vi "My JKI State Machine Module.vi"(7 "Module Name":string="M1") -> ()   [LabVIEW 2017, in "CSM Example echo DQMH.lvlib"]
doc: "------------- lvcsm -------------\n[CSMStates]\nItem 0 = \"Event Structure\"\nItem 1 = \"Idle\"\nItem 2 = \"Target Timeout Error\"\nItem 3 = \"Target Error\"\nItem 4 = \"Initialize Core Data\"\nItem 5 = \"VI Reference\"\nItem 6 = \"Error Handler\"\nItem 7 = \"Exit\"\nItem 8 = \"Data: Initialize\"\nItem 9 = \"Data: Cleanup\"\nItem 10 = \"UI: Initialize\"\nItem 11 = \"UI: Cursor Set\"\nItem 12 = \"UI: Front Panel State\"\nItem 13 = \"Macro: Initialize\"\nItem 14 = \"Macro: Exit\"\nItem 15 = \"New Category: 1\"\nItem 16 = \"New Category: 2\"\nItem 17 = \"Test: Do Something\"\nItem 18 = \"Test: Do Something Else\"\nItem 19 = \"Test: Do Something Else and Wait for Reply\"\n\n[CSMStatus]\nItem 0 = \"Test: Do Something Else@Event Structure\"\nItem 1 = \"Test: Do Something Else@Idle\""
uses:
  CSM Example echo DQMH.lvlib
  <vilib>/ErrorRing/Error Ring.xnode
  user.lib/_NEVSTOP/Communicable State Machine(CSM)/Communicable State Machine.lvlib
panel:
  out "Status":string
  out "error out":errorcluster
  in  "Simulate  Error":bool
  out "X":dbl
  in  "Do Something Else <Replace Me>":bool
  in  "Do Something <Replace Me>":bool
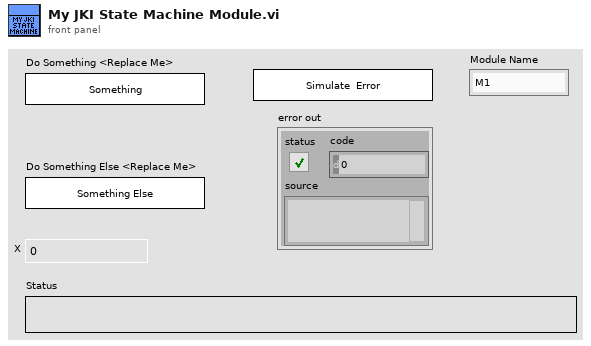
[diagram p1: front panel]
types:
  T1 = enum32{"Invalid", "Standard", "Closed", "Hidden", "Minimized", "Maximized"}
  T2 = enum32{"invalid app kind", "Development System", "Run Time System", "Student Edition", "Embedded LabVIEW", "Evaluation", "Custom"}
  T3 = cluster{"Core":cluster{"Current VI Reference":refnum<vi>, "Close Panel on Exit?":bool}, "Your Boolean data":bool, "Your string data":string}
  T4 = cluster{"Current VI Reference":refnum<vi>, "Close Panel on Exit?":bool}
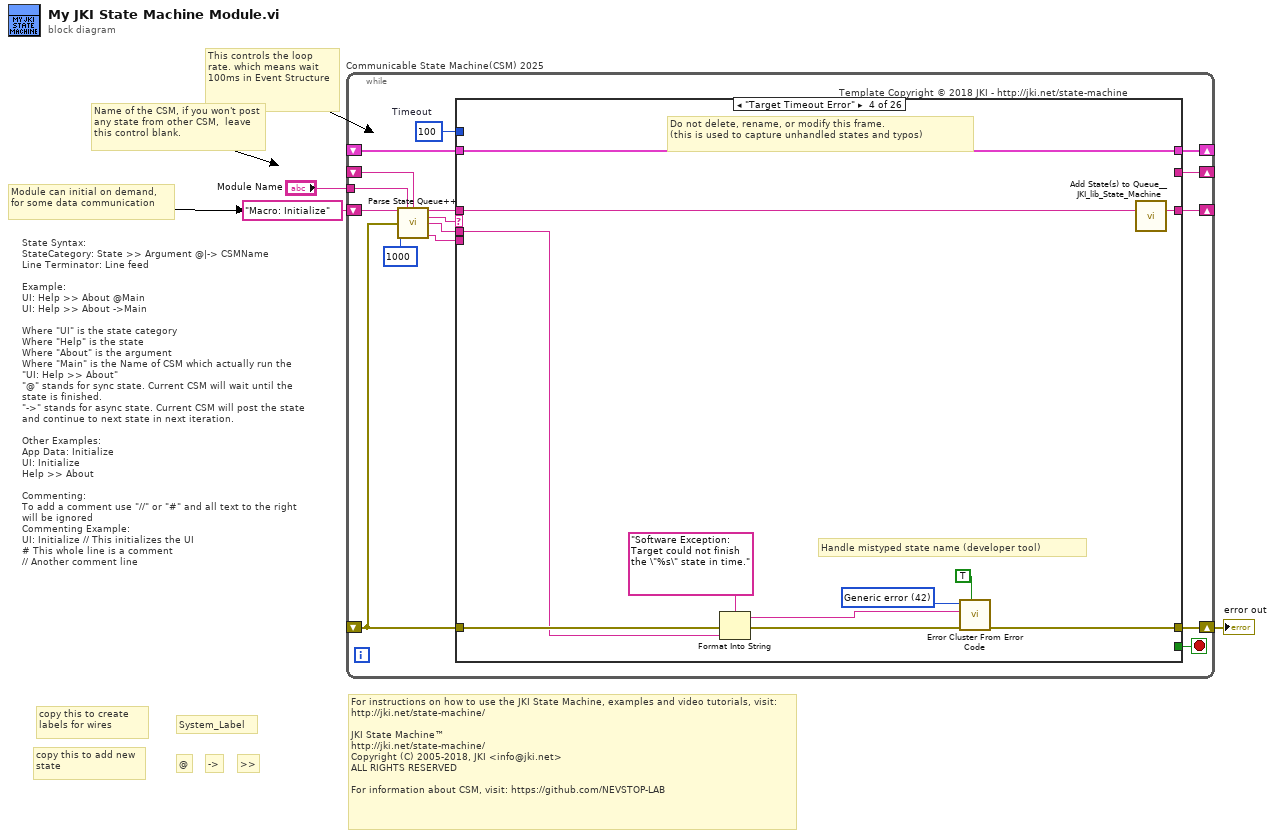
[diagram p0: block diagram]
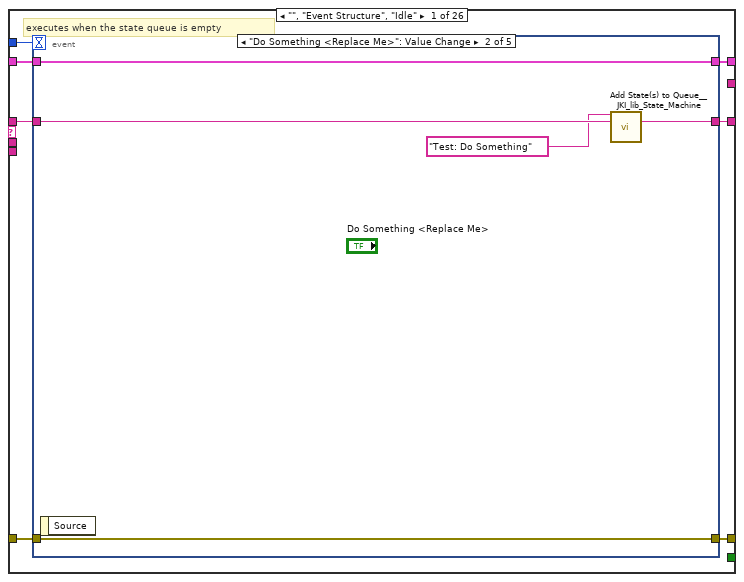
[diagram p2: hidden frame]
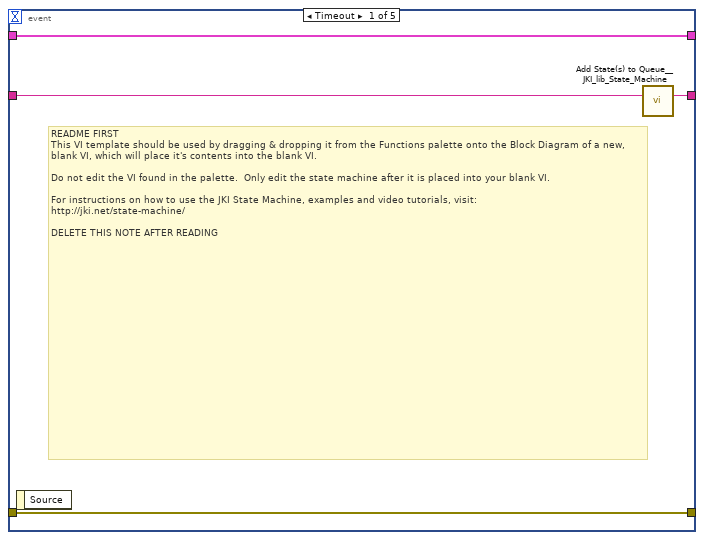
[diagram p3: hidden frame]
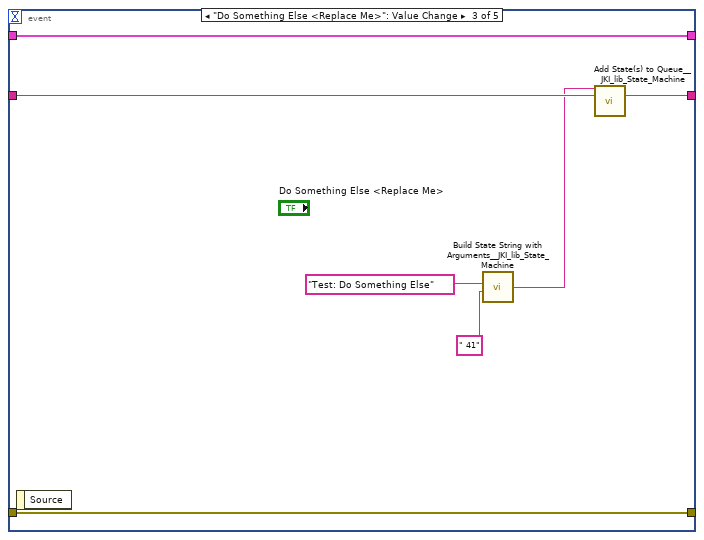
[diagram p4: hidden frame]
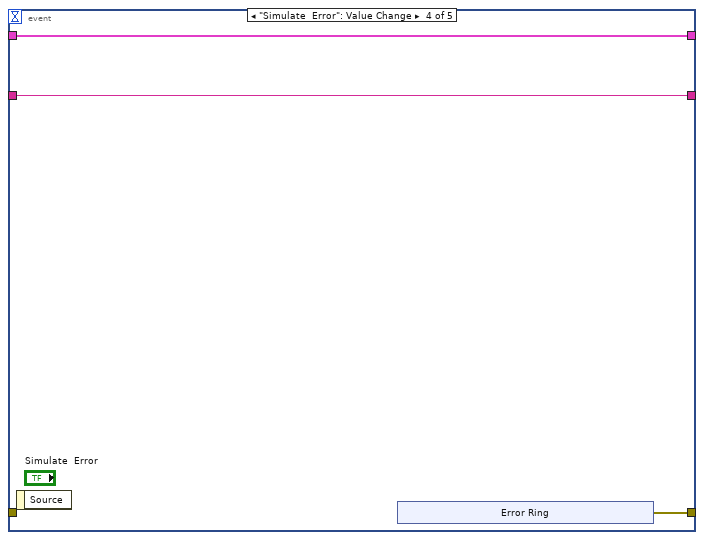
[diagram p5: hidden frame]
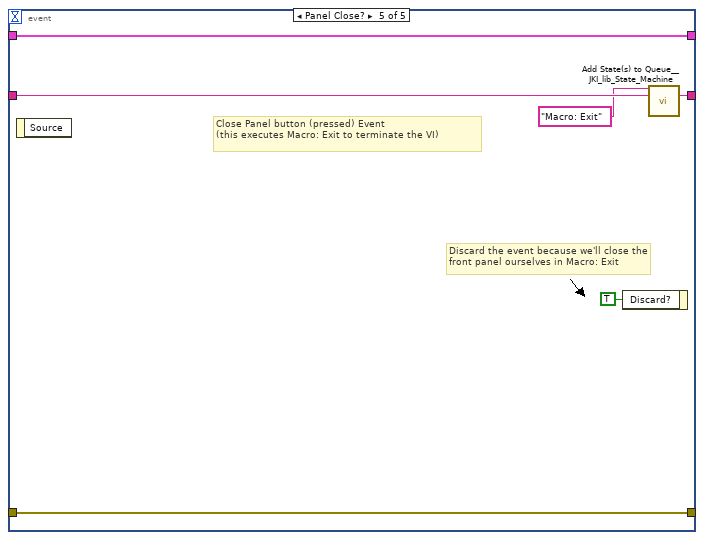
[diagram p6: hidden frame]
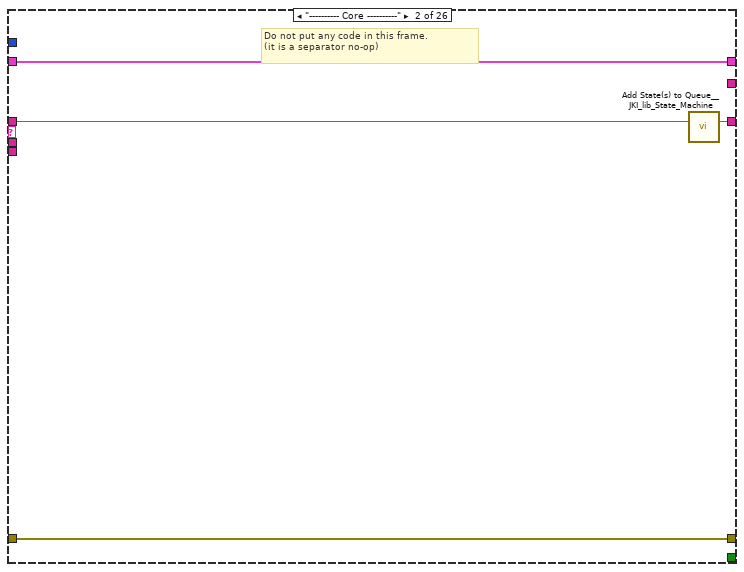
[diagram p7: hidden frame]
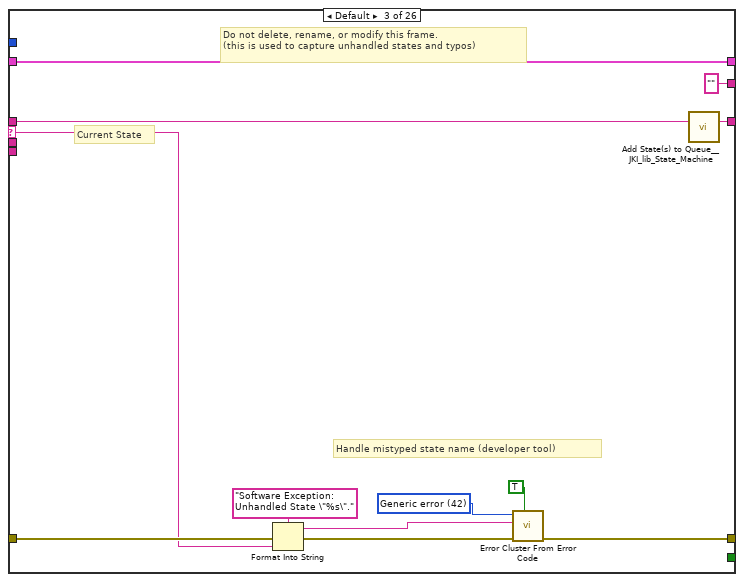
[diagram p8: hidden frame]
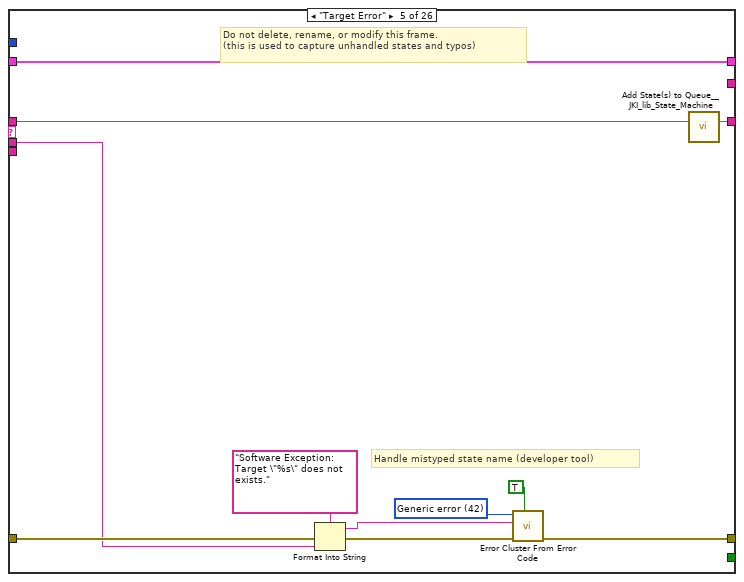
[diagram p9: hidden frame]
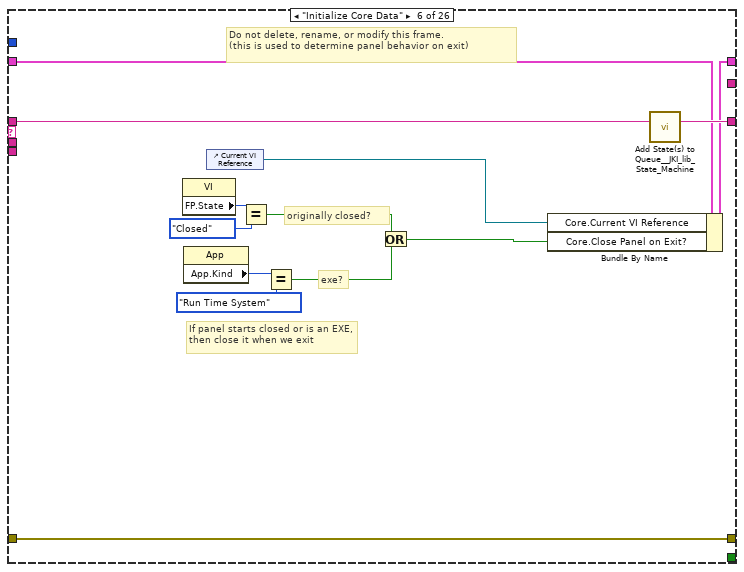
[diagram p10: hidden frame]
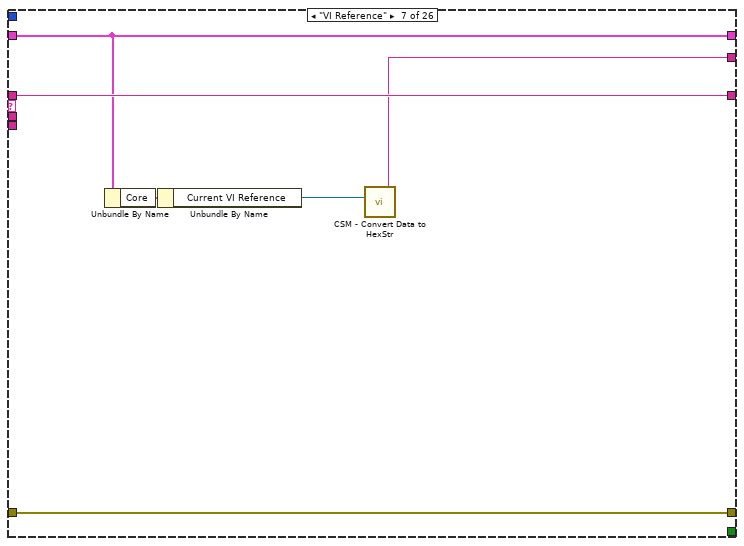
[diagram p11: hidden frame]
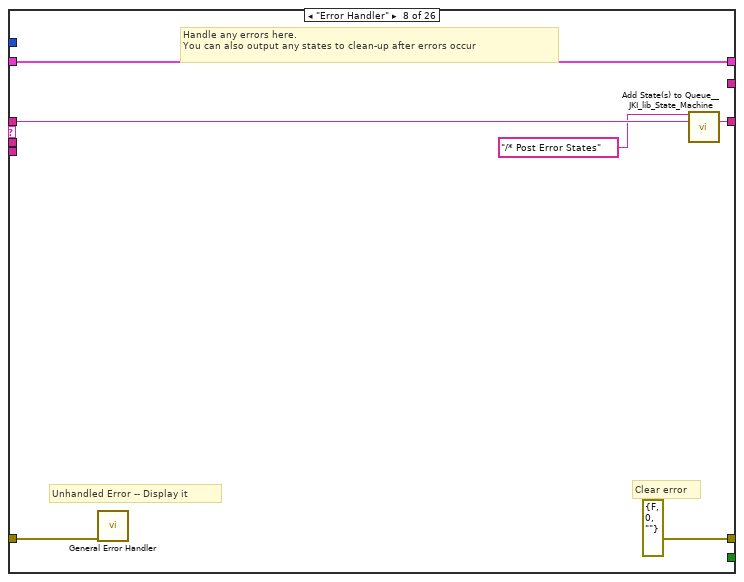
[diagram p12: hidden frame]
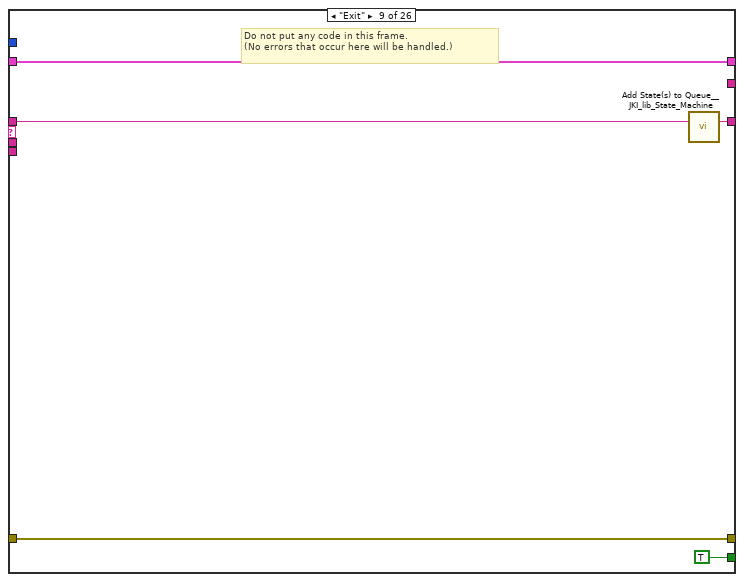
[diagram p13: hidden frame]
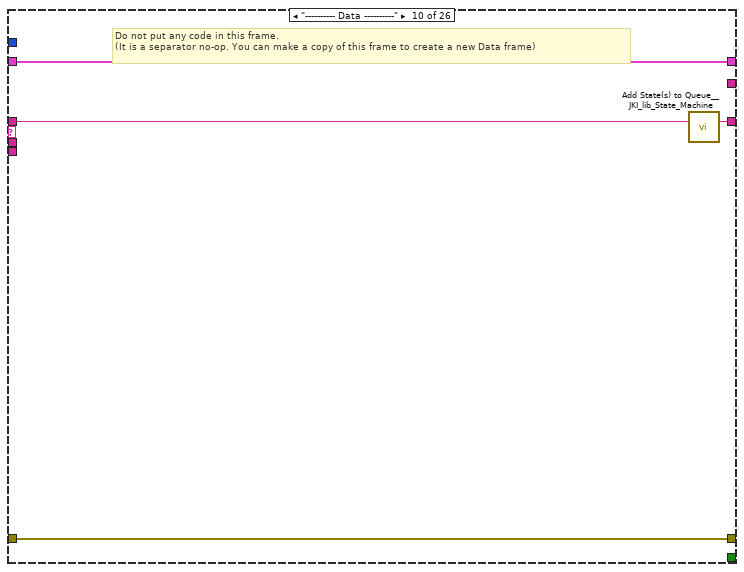
[diagram p14: hidden frame]
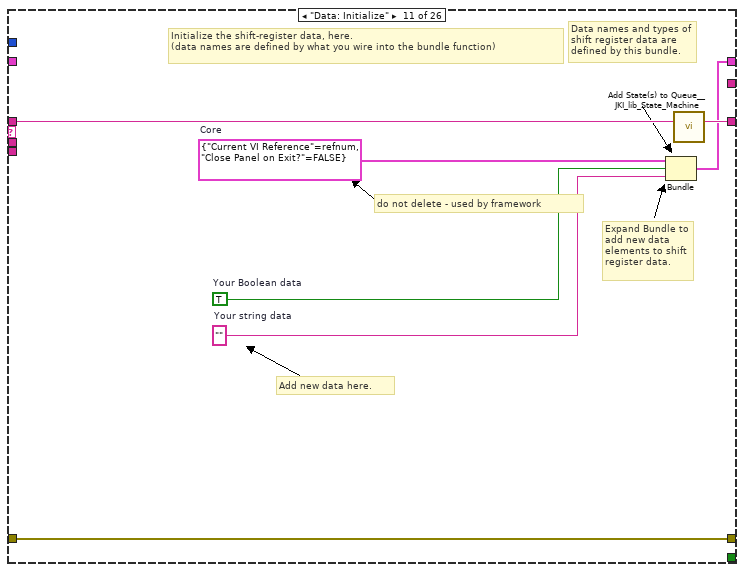
[diagram p15: hidden frame]
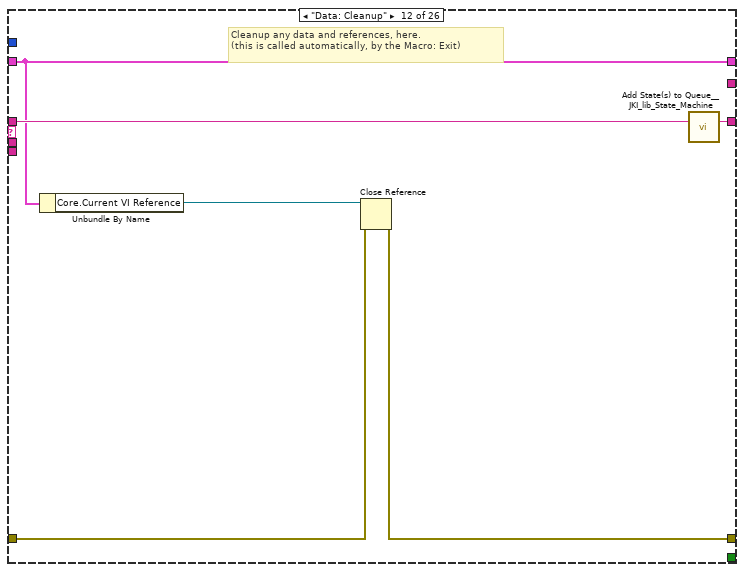
[diagram p16: hidden frame]
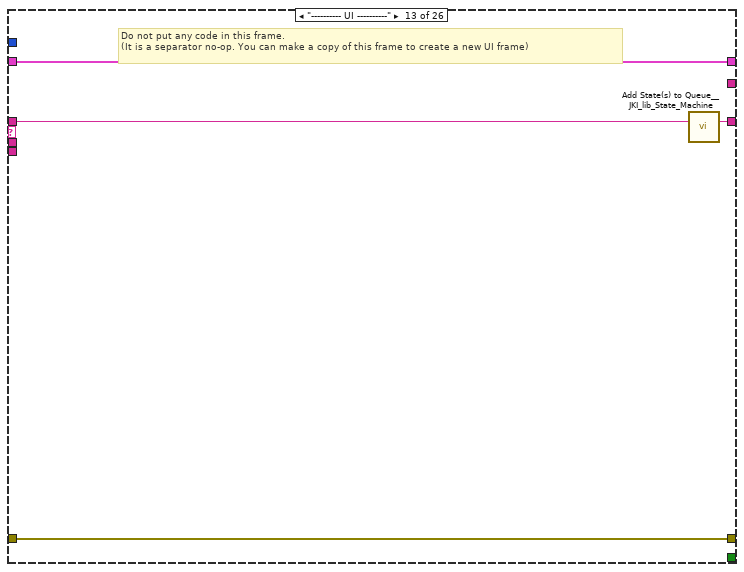
[diagram p17: hidden frame]
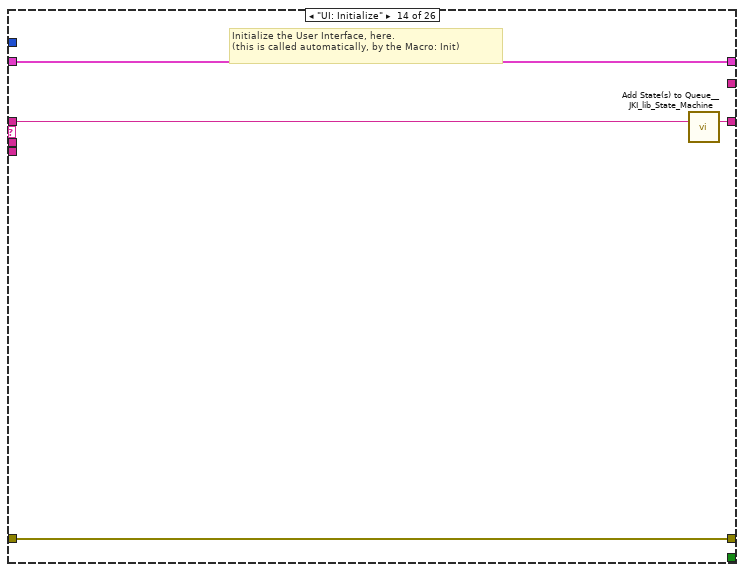
[diagram p18: hidden frame]
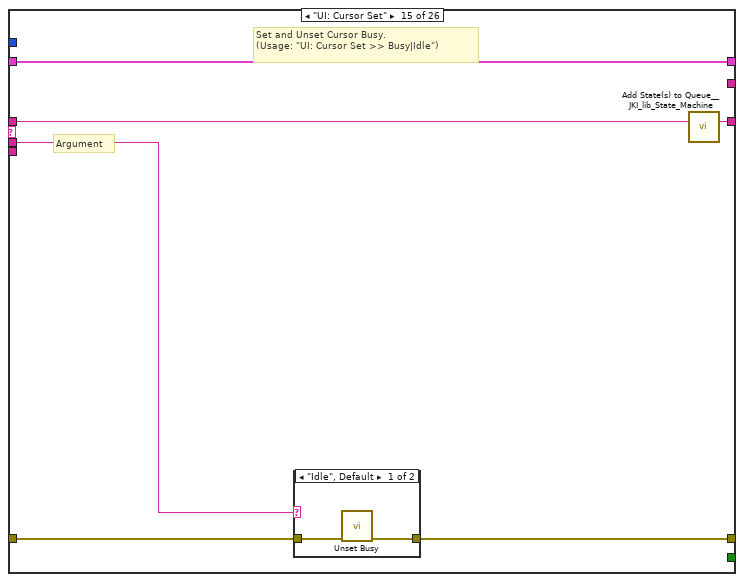
[diagram p19: hidden frame]
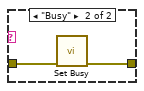
[diagram p20: hidden frame]
diagram:
  # "For instructions on how to use the JKI State Machine, examples and video tutorials, visit: http://jki.net/state-machine/\n\nJKI State Machine™\nhttp://jki.net/state-machine/\nCopyright (C) 2005-2018, JKI <info@jki.net>\nALL RIGHTS RESERVED\n\nFor information about CSM, visit: https://github.com/NEVSTOP-LAB"
  # "copy this to add new state"
  # ">>"
  # "->"
  # "@"
  # "State Syntax:\nStateCategory: State >> Argument @|-> CSMName\nLine Terminator: Line feed\n\nExample:\nUI: Help >> About @Main\nUI: Help >> About ->Main\n\nWhere \"UI\" is the state category\nWhere \"Help\" is the state\nWhere \"About\" is the argument\nWhere \"Main\" is the Name of CSM which actually run the \"UI: Help >> About\"\n\"@\" stands for sync state. Current CSM will wait until the state is finished.\n\"->\" stands for async state. Current CSM will post the state and continue to next state in next iteration.\n\nOther Examples:\nApp Data: Initialize\nUI: Initialize\nHelp >> About\n\nCommenting:\nTo add a comment use \"//\" or \"#\" and all text to the right will be ignored\nCommenting Example:\nUI: Initialize // This initializes the UI\n# This whole line is a comment\n// Another comment line"
  # "copy this to create labels for wires"
  # "System_Label"
  # "Module can initial on demand,\nfor some data communication"
  # "Name of the CSM, if you won't post any state from other CSM,  leave this control blank."
  # "This controls the loop rate. which means wait 100ms in Event Structure"
  n1 = while "Communicable State Machine(CSM) 2025" {
    shift-right: [w14] -> _
    shift-left: _ -> [w13]
    shift-right: [w17] -> w1
    shift-left: _ -> [w11]
    shift-right: [w16] -> _
    shift-left: "Macro: Initialize" ("States Out") -> [w18]
    tunnel: "Module Name" -> [w7]
    shift-right: [w4] -> _
    shift-left: _ -> [w5]
    stop <- w15 stop-if-true
    w12 = 100  # Timeout
    # "Template Copyright © 2018 JKI - http://jki.net/state-machine"
    n2 = call "Parse State Queue++.vi"("State Queue"=w18, "Name (\"\" to Use UUID)"=w7, "Response Arguments"=w5, "Previous Error"=w11, "Response Timeout (-2 Use Global Settings)"=1000 ("Response Timeout(1000ms)")) -> ("Remaining States"=w19:string, "Current State"=w10:string, "Arguments"=w9:string, ">> Source CSM >>"=w8:string)  [unwired: 5 in, 2 out]
    n3 = case shown="\"Target Timeout Error\"" w10 {
      selector: w10 -> [_ _ w62 _ _ _ _ _ _ _ _ _ _ _ _ _ _ _ _ _ _ _ _ _ _ _]
      tunnel: w19 -> [w26 w60 w66 w77 w88 w107 w112 w119 w124 w128 w135 w141 w145 w149 w155 w166 w235 w240 w250 w254 w258 w262 w266 w277 w291 w307]
      tunnel: w9 -> [_ _ _ w73 w84 _ _ _ _ _ _ _ _ _ w150 w160 _ _ _ _ _ _ _ _ w281 w296]
      tunnel: w13 -> [w24 w57 w64 w75 w86 w100 w111 w116 w122 w125 _ w136 w142 w147 w153 w162 w232 w237 w247 w251 w255 w259 w263 w276 w290 w306]
      tunnel: [w23 w58 w68 w79 w90 w104 w113 errorcluster {"status"=FALSE, "code"=0, "source"=""} ("error out") w121 w126 w132 w137 w143 w146 w151 w163 w233 w238 w248 w252 w256 w260 w264 w278 w292 w308] -> w17
      tunnel: w11 -> [w22 w58 w67 w78 w89 w104 w113 w115 w121 w126 w132 w138 w143 w146 w152 w164 w233 w238 w248 w252 w256 w260 w264 w278 w292 w308]
      tunnel: [w25 w59 w65 w76 w87 w106 w112 w118 w123 w127 w134 w140 w144 w148 w154 w165 w234 w239 w249 w253 w257 w261 w265 w277 w291 w307] -> w16
      tunnel: [_ _ _ _ _ _ _ _ TRUE _ _ _ _ _ _ _ _ _ _ _ _ _ _ _ _ _] -> w15
      tunnel: [w21 w57 w64 w75 w86 w105 w111 w116 w122 w125 w133 w136 w142 w147 w153 w162 w232 w237 w247 w251 w255 w259 w263 w276 w290 w306] -> w14
      tunnel: w12 -> [w20 _ _ _ _ _ _ _ _ _ _ _ _ _ _ _ _ _ _ _ _ _ _ _ _ _]
      tunnel: w8 -> [_ _ _ _ _ _ _ _ _ _ _ _ _ _ _ _ _ _ _ _ _ _ _ w268 w283 w299]
      tunnel: [_ _ "" _ _ _ w108 _ _ _ _ _ _ _ _ _ _ _ _ _ _ _ _ w267 w279 w293] -> w4
      frame "", "Event Structure", "Idle" {
        # "executes when the state queue is empty"
        n4 = event shown="[1] \"Do Something <Replace Me>\": Value Change" {
          selector: _ -> [_ _ _ _ _]
          dyn-events: _ -> [_ _ _ _ _]
          timeout: w20 -> [_ _ _ _ _]
          tunnel: w26 -> [w30 w35 w42 w44 w56]
          tunnel: [w29 w34 w41 w44 w55] -> w25
          tunnel: w24 -> [w27 w33 w40 w45 w53]
          tunnel: [w28 w31 w39 w43 w54] -> w23
          tunnel: w22 -> [w28 w31 w39 _ w54]
          tunnel: [w27 w33 w40 w45 w53] -> w21
          event Timeout {
            # "README FIRST\nThis VI template should be used by dragging & dropping it from the Functions palette onto the Block Diagram of a new, blank VI, which will place it's contents into the blank VI.\n\nDo not edit the VI found in the palette.  Only edit the state machine after it is placed into your blank VI.\n\nFor instructions on how to use the JKI State Machine, examples and video tutorials, visit:\nhttp://jki.net/state-machine/\n\nDELETE THIS NOTE AFTER READING"
            n5 = event-data() -> ()  [unwired: 1 in, 1 out]
            n6 = call <vilib>:"Add State(s) to Queue__JKI_lib_State_Machine.vi"("State(s) in (\"\")"=w30) -> ("States Out"=w29:string)  [unwired: 14 in]
          }
          event "Do Something <Replace Me>": Value Change {
            n7 = event-data() -> ()  [unwired: 1 in, 1 out]
            n8 = call <vilib>:"Add State(s) to Queue__JKI_lib_State_Machine.vi"("State(s) in Front (\"\")"="Test: Do Something" ("State(s) in Front (\"\")"), "State(s) in (\"\")"=w35) -> ("States Out"=w34:string)  [unwired: 13 in]
          }
          event "Do Something Else <Replace Me>": Value Change {
            n9 = event-data() -> ()  [unwired: 1 in, 1 out]
            n10 = call <vilib>:"Build State String with Arguments__JKI_lib_State_Machine.vi"("Arguments (\"\")"=" 41" ("Arguments (\"\")"), "State"="Test: Do Something Else" ("State(s) in Front (\"\")")) -> ("State with Arguments"=w37:string)  [unwired: 4 in]
            n11 = call <vilib>:"Add State(s) to Queue__JKI_lib_State_Machine.vi"("State(s) in Front (\"\")"=w37, "State(s) in (\"\")"=w42) -> ("States Out"=w41:string)  [unwired: 13 in]
          }
          event "Simulate  Error": Value Change {
            n12 = event-data() -> ()  [unwired: 1 in, 1 out]
            n13 = xnode "Error Ring"() -> ("error out"=w43:errorcluster)
          }
          event Panel Close? {
            # "Discard the event because we'll close the front panel ourselves in Macro: Exit"
            # "Close Panel button (pressed) Event\n(this executes Macro: Exit to terminate the VI)"
            n14 = event-data() -> ()  [unwired: 1 in, 1 out]
            n15 = event-data("Discard?"=TRUE) -> ()  [unwired: 1 in, 1 out]
            n16 = call <vilib>:"Add State(s) to Queue__JKI_lib_State_Machine.vi"("State(s) in Front (\"\")"="Macro: Exit", "State(s) in (\"\")"=w56) -> ("States Out"=w55:string)  [unwired: 13 in]
          }
        }
      }
      frame "---------- Core ----------" {
        # "Do not put any code in this frame.\n(it is a separator no-op)"
        n17 = call <vilib>:"Add State(s) to Queue__JKI_lib_State_Machine.vi"("State(s) in (\"\")"=w60) -> ("States Out"=w59:string)  [unwired: 14 in]
      }
      frame Default {
        w71 = 42 items=["No error", "Argument error", "Memory is full", "Out of zone", "End of file", "File already open", "Generic file I/O error", "File not found", "File permission error", "Disk is full", "Duplicate path", "Too many files open", "System feature not enabled", "Resource file not found", "Cannot add resource", "Resource not found", "Image not found", "Image memory error", "Pen does not exist", "Config type invalid", "Config token not found", "Config parse error", "Config memory error", "Bad external code format", "Bad external code offset", "External code not present", "Null window", "Destroy window error", "Null menu", "Print aborted", "Bad print record", "Print driver error", "Windows error during printing", "Memory error during printing", "Print dialog error", "Generic print error", "Invalid device refnum", "Device not found", "Device parameter error", "Device unit error", "Cannot open device", "Device call aborted", "Generic error", "Cancelled by user", "Object ID too low", "Object ID too high", "Object not in heap", "Unknown heap", "Unknown object (invalid DefProc)", "Unknown object (DefProc not in table)", "Message out of range", "Invalid (null) method", "Unknown message", "Manager call not supported", "Bad address", "Network operation in progress", "Network operation timed out", "Connection is busy", "Network attribute not supported", "Network error", "Address in use", "System out of memory", "Connection aborted", "Connection refused", "Not connected", "Already connected", "Connection closed", "Initialization error (interapplication manager)", "Bad occurrence", "Wait on unbound occurrence handler", "Occurrence queue overflow", "Datalog type conflict", "Unused", "Unrecognized type (interapplication manager)", "Memory corrupt", "Failed to make temporary DLL", "Old CIN version", "Drag socket not found", "Failed to load drop-object", "Failed to register OLE object", "Failed to release OLE object", "Format specifier type mismatch", "Unknown format specifier", "Too few format specifiers", "Too many format specifiers", "Scan failed", "Newer CIN version", "Error converting to variant", "Runtime menu error", "Password tampered", "Variant attribute not found", "Incompatible variant data type", "Event data is not available", "Event Store is not present", "Occurrence is not found", "Event Queue is not created", "Event info is not available", "Refnum passed is NULL", "Error retrieving Class GUID", "Error retrieving CoClass GUID", "Error retrieving TypeLib GUID.", "Bad built application magic bytes.", "Specific driver is different from the specific driver associated with the Logical Name.", "There is no session opened to the class driver.", "Max Error", "MAX - Error with config objects", "MAX - Error loading configuration", "MAX - Group not supported"]
        # "Current State"
        # "Do not delete, rename, or modify this frame.\n(this is used to capture unhandled states and typos)"
        # "Handle mistyped state name (developer tool)"
        n18 = Format Into String(format string="Software Exception: Unhandled State \"%s\"." ("message"), error in=w67, w62) -> (resulting string=w70:string, error out=w69:errorcluster)  [unwired: 1 in]
        n19 = call <vilib>:"Error Cluster From Error Code.vi"("show call chain? (False)"=TRUE, "error in (no error)"=w69, "error message (\"\")"=w70, "error code (0)"=w71) -> ("error out"=w68:errorcluster)  [unwired: 5 in]
        n20 = call <vilib>:"Add State(s) to Queue__JKI_lib_State_Machine.vi"("State(s) in (\"\")"=w66) -> ("States Out"=w65:string)  [unwired: 14 in]
      }
      frame "Target Timeout Error" {
        w82 = 42 items=["No error", "Argument error", "Memory is full", "Out of zone", "End of file", "File already open", "Generic file I/O error", "File not found", "File permission error", "Disk is full", "Duplicate path", "Too many files open", "System feature not enabled", "Resource file not found", "Cannot add resource", "Resource not found", "Image not found", "Image memory error", "Pen does not exist", "Config type invalid", "Config token not found", "Config parse error", "Config memory error", "Bad external code format", "Bad external code offset", "External code not present", "Null window", "Destroy window error", "Null menu", "Print aborted", "Bad print record", "Print driver error", "Windows error during printing", "Memory error during printing", "Print dialog error", "Generic print error", "Invalid device refnum", "Device not found", "Device parameter error", "Device unit error", "Cannot open device", "Device call aborted", "Generic error", "Cancelled by user", "Object ID too low", "Object ID too high", "Object not in heap", "Unknown heap", "Unknown object (invalid DefProc)", "Unknown object (DefProc not in table)", "Message out of range", "Invalid (null) method", "Unknown message", "Manager call not supported", "Bad address", "Network operation in progress", "Network operation timed out", "Connection is busy", "Network attribute not supported", "Network error", "Address in use", "System out of memory", "Connection aborted", "Connection refused", "Not connected", "Already connected", "Connection closed", "Initialization error (interapplication manager)", "Bad occurrence", "Wait on unbound occurrence handler", "Occurrence queue overflow", "Datalog type conflict", "Unused", "Unrecognized type (interapplication manager)", "Memory corrupt", "Failed to make temporary DLL", "Old CIN version", "Drag socket not found", "Failed to load drop-object", "Failed to register OLE object", "Failed to release OLE object", "Format specifier type mismatch", "Unknown format specifier", "Too few format specifiers", "Too many format specifiers", "Scan failed", "Newer CIN version", "Error converting to variant", "Runtime menu error", "Password tampered", "Variant attribute not found", "Incompatible variant data type", "Event data is not available", "Event Store is not present", "Occurrence is not found", "Event Queue is not created", "Event info is not available", "Refnum passed is NULL", "Error retrieving Class GUID", "Error retrieving CoClass GUID", "Error retrieving TypeLib GUID.", "Bad built application magic bytes.", "Specific driver is different from the specific driver associated with the Logical Name.", "There is no session opened to the class driver.", "Max Error", "MAX - Error with config objects", "MAX - Error loading configuration", "MAX - Group not supported"]
        # "Do not delete, rename, or modify this frame.\n(this is used to capture unhandled states and typos)"
        # "Handle mistyped state name (developer tool)"
        n21 = Format Into String(format string="Software Exception: Target could not finish the \"%s\" state in time." ("message"), error in=w78, w73) -> (resulting string=w81:string, error out=w80:errorcluster)  [unwired: 1 in]
        n22 = call <vilib>:"Error Cluster From Error Code.vi"("show call chain? (False)"=TRUE, "error in (no error)"=w80, "error message (\"\")"=w81, "error code (0)"=w82) -> ("error out"=w79:errorcluster)  [unwired: 5 in]
        n23 = call <vilib>:"Add State(s) to Queue__JKI_lib_State_Machine.vi"("State(s) in (\"\")"=w77) -> ("States Out"=w76:string)  [unwired: 14 in]
      }
      frame "Target Error" {
        w93 = 42 items=["No error", "Argument error", "Memory is full", "Out of zone", "End of file", "File already open", "Generic file I/O error", "File not found", "File permission error", "Disk is full", "Duplicate path", "Too many files open", "System feature not enabled", "Resource file not found", "Cannot add resource", "Resource not found", "Image not found", "Image memory error", "Pen does not exist", "Config type invalid", "Config token not found", "Config parse error", "Config memory error", "Bad external code format", "Bad external code offset", "External code not present", "Null window", "Destroy window error", "Null menu", "Print aborted", "Bad print record", "Print driver error", "Windows error during printing", "Memory error during printing", "Print dialog error", "Generic print error", "Invalid device refnum", "Device not found", "Device parameter error", "Device unit error", "Cannot open device", "Device call aborted", "Generic error", "Cancelled by user", "Object ID too low", "Object ID too high", "Object not in heap", "Unknown heap", "Unknown object (invalid DefProc)", "Unknown object (DefProc not in table)", "Message out of range", "Invalid (null) method", "Unknown message", "Manager call not supported", "Bad address", "Network operation in progress", "Network operation timed out", "Connection is busy", "Network attribute not supported", "Network error", "Address in use", "System out of memory", "Connection aborted", "Connection refused", "Not connected", "Already connected", "Connection closed", "Initialization error (interapplication manager)", "Bad occurrence", "Wait on unbound occurrence handler", "Occurrence queue overflow", "Datalog type conflict", "Unused", "Unrecognized type (interapplication manager)", "Memory corrupt", "Failed to make temporary DLL", "Old CIN version", "Drag socket not found", "Failed to load drop-object", "Failed to register OLE object", "Failed to release OLE object", "Format specifier type mismatch", "Unknown format specifier", "Too few format specifiers", "Too many format specifiers", "Scan failed", "Newer CIN version", "Error converting to variant", "Runtime menu error", "Password tampered", "Variant attribute not found", "Incompatible variant data type", "Event data is not available", "Event Store is not present", "Occurrence is not found", "Event Queue is not created", "Event info is not available", "Refnum passed is NULL", "Error retrieving Class GUID", "Error retrieving CoClass GUID", "Error retrieving TypeLib GUID.", "Bad built application magic bytes.", "Specific driver is different from the specific driver associated with the Logical Name.", "There is no session opened to the class driver.", "Max Error", "MAX - Error with config objects", "MAX - Error loading configuration", "MAX - Group not supported"]
        # "Do not delete, rename, or modify this frame.\n(this is used to capture unhandled states and typos)"
        # "Handle mistyped state name (developer tool)"
        n24 = Format Into String(format string="Software Exception: Target \"%s\" does not exists." ("message"), error in=w89, w84) -> (resulting string=w92:string, error out=w91:errorcluster)  [unwired: 1 in]
        n25 = call <vilib>:"Error Cluster From Error Code.vi"("show call chain? (False)"=TRUE, "error in (no error)"=w91, "error message (\"\")"=w92, "error code (0)"=w93) -> ("error out"=w90:errorcluster)  [unwired: 5 in]
        n26 = call <vilib>:"Add State(s) to Queue__JKI_lib_State_Machine.vi"("State(s) in (\"\")"=w88) -> ("States Out"=w87:string)  [unwired: 14 in]
      }
      frame "Initialize Core Data" {
        # "Do not delete, rename, or modify this frame.\n(this is used to determine panel behavior on exit)"
        # "originally closed?"
        # "exe?"
        # "If panel starts closed or is an EXE, then close it when we exit"
        n27 = property class="VI"() -> ("FP.State"=w97:T1)  [unwired: 2 in, 2 out]
        n28 = property class="App"() -> ("App.Kind"=w103:T2)  [unwired: 2 in, 2 out]
        n29 = control-ref of="Current VI Reference"() -> (w98:refnum<vi>)
        n30 = Equal?(x=w97, y=T1."Closed" ("Front Panel Window:State")) -> (x = y?=w95:bool)
        n31 = Equal?(x=w103, y=T2."Run Time System" ("Application:Kind")) -> (x = y?=w101:bool)
        n32 = Or(x=w95, y=w101) -> (x .or. y?=w99:bool)
        n33 = Bundle By Name(cluster=w100, "Core.Current VI Reference"=w98, "Core.Close Panel on Exit?"=w99) -> (w105:T3)
        n34 = call <vilib>:"Add State(s) to Queue__JKI_lib_State_Machine.vi"("State(s) in (\"\")"=w107) -> ("States Out"=w106:string)  [unwired: 14 in]
      }
      frame "VI Reference" {
        n35 = Unbundle By Name(w111) -> ("Core"=w110:T4)
        n36 = Unbundle By Name(w110) -> ("Current VI Reference"=w109:refnum<vi>)
        n37 = call "CSM - Convert Data to HexStr.vi"("Variant"=w109) -> ("HEX String (0-9,A-F)"=w108:string)  [unwired: 8 in]
      }
      frame "Error Handler" {
        # "Unhandled Error -- Display it"
        # "Handle any errors here.\nYou can also output any states to clean-up after errors occur"
        # "Clear error"
        n38 = call <vilib>:"General Error Handler.vi"("error in (no error)"=w115) -> ()  [unwired: 10 in, 5 out]
        n39 = call <vilib>:"Add State(s) to Queue__JKI_lib_State_Machine.vi"("State(s) in Front (\"\")"="/* Post Error States", "State(s) in (\"\")"=w119) -> ("States Out"=w118:string)  [unwired: 13 in]
      }
      frame "Exit" {
        # "Do not put any code in this frame.\n(No errors that occur here will be handled.)"
        n40 = call <vilib>:"Add State(s) to Queue__JKI_lib_State_Machine.vi"("State(s) in (\"\")"=w124) -> ("States Out"=w123:string)  [unwired: 14 in]
      }
      frame "---------- Data ----------" {
        # "Do not put any code in this frame.\n(It is a separator no-op. You can make a copy of this frame to create a new Data frame)"
        n41 = call <vilib>:"Add State(s) to Queue__JKI_lib_State_Machine.vi"("State(s) in (\"\")"=w128) -> ("States Out"=w127:string)  [unwired: 14 in]
      }
      frame "Data: Initialize" {
        w129 = T4 {"Current VI Reference"=refnum, "Close Panel on Exit?"=FALSE}  # Core
        w131 = TRUE  # Your Boolean data
        w130 = ""  # Your string data
        # "do not delete - used by framework"
        # "Expand Bundle to add new data elements to shift register data."
        # "Add new data here."
        # "Data names and types of shift register data are defined by this bundle."
        # "Initialize the shift-register data, here.\n(data names are defined by what you wire into the bundle function)"
        n42 = Bundle("Core"=w129, "Your Boolean data"=w131, "Your string data"=w130) -> (w133:T3)  [unwired: 1 in]
        n43 = call <vilib>:"Add State(s) to Queue__JKI_lib_State_Machine.vi"("State(s) in (\"\")"=w135) -> ("States Out"=w134:string)  [unwired: 14 in]
      }
      frame "Data: Cleanup" {
        # "Cleanup any data and references, here.\n(this is called automatically, by the Macro: Exit)"
        n44 = Unbundle By Name(w136) -> ("Core.Current VI Reference"=w139:refnum<vi>)
        n45 = Close Reference(reference=w139, error in (no error)=w138) -> (error out=w137:errorcluster)
        n46 = call <vilib>:"Add State(s) to Queue__JKI_lib_State_Machine.vi"("State(s) in (\"\")"=w141) -> ("States Out"=w140:string)  [unwired: 14 in]
      }
      frame "---------- UI ----------" {
        # "Do not put any code in this frame.\n(It is a separator no-op. You can make a copy of this frame to create a new UI frame)"
        n47 = call <vilib>:"Add State(s) to Queue__JKI_lib_State_Machine.vi"("State(s) in (\"\")"=w145) -> ("States Out"=w144:string)  [unwired: 14 in]
      }
      frame "UI: Initialize" {
        # "Initialize the User Interface, here.\n(this is called automatically, by the Macro: Init)"
        n48 = call <vilib>:"Add State(s) to Queue__JKI_lib_State_Machine.vi"("State(s) in (\"\")"=w149) -> ("States Out"=w148:string)  [unwired: 14 in]
      }
      frame "UI: Cursor Set" {
        # "Argument"
        # "Set and Unset Cursor Busy.\n(Usage: \"UI: Cursor Set >> Busy|Idle\")"
        n49 = case shown="\"Idle\", Default" w150 {
          tunnel: w152 -> [w157 w159]
          tunnel: [w156 w158] -> w151
          frame "Idle", Default {
            n50 = call <vilib>:"Unset Busy.vi"("error in (no error)"=w157) -> ("error out"=w156:errorcluster)  [unwired: 10 in]
          }
          frame "Busy" {
            n51 = call <vilib>:"Set Busy.vi"("error in (no error)"=w159) -> ("error out"=w158:errorcluster)  [unwired: 9 in, 1 out]
          }
        }
        n52 = call <vilib>:"Add State(s) to Queue__JKI_lib_State_Machine.vi"("State(s) in (\"\")"=w155) -> ("States Out"=w154:string)  [unwired: 14 in]
      }
      frame "UI: Front Panel State" {
        # "Argument"
        # "Set Front Panel Open or Closed\n(Usage: \"UI: Front Panel State >> Open|Close\")"
        n53 = Unbundle By Name(w162) -> ("Core.Current VI Reference"=w161:refnum<vi>)
        n54 = case shown="\"Minimize\", \"Minimized\"" w160 {
          tunnel: w164 -> [w172 w187 w198 w211 w224]
          tunnel: [w174 w188 w200 w213 w226] -> w163
          tunnel: w161 -> [w173 w185 w199 w212 w225]
          frame "Open", "Standard", Default {
            w167 = T1."Standard" ("State")
            n55 = property class="VI"(reference=w173, error in=w172) -> (reference out=w170:refnum<vi>, error out=w171:errorcluster, "FP.State"=w169:T1)
            n56 = Not Equal?(x=w169, y=w167) -> (x != y?=w168:bool)
            n57 = case shown="True" w168 {
              tunnel: [w178 w180] -> w174
              tunnel: w171 -> [w177 w180]
              tunnel: w170 -> [w176 _]
              tunnel: w167 -> [w175 _]
              frame True {
                n58 = invoke class="VI" method="FP.Open"(reference=w176, error in=w177, "Activate"=TRUE, "State"=w175) -> (error out=w178:errorcluster)  [unwired: 1 in, 4 out]
              }
              frame False {
              }
            }
          }
          frame "Close", "Closed" {
            n59 = property class="VI"(reference=w185, error in=w187) -> (reference out=w184:refnum<vi>, error out=w186:errorcluster, "FP.State"=w182:T1)
            n60 = Not Equal?(x=w182, y=T1."Closed" ("Front Panel Window:State")) -> (x != y?=w181:bool)
            n61 = case shown="True" w181 {
              tunnel: [w189 w192] -> w188
              tunnel: w186 -> [w189 w191]
              tunnel: w184 -> [_ w190]
              frame False {
              }
              frame True {
                n62 = invoke class="VI" method="FP.Close"(reference=w190, error in=w191) -> (error out=w192:errorcluster)  [unwired: 1 in, 2 out]
              }
            }
          }
          frame "Hidden", "Hide" {
            w193 = T1."Hidden" ("State")
            n63 = property class="VI"(reference=w199, error in=w198) -> (reference out=w196:refnum<vi>, error out=w197:errorcluster, "FP.State"=w195:T1)
            n64 = Not Equal?(x=w195, y=w193) -> (x != y?=w194:bool)
            n65 = case shown="True" w194 {
              tunnel: [w204 w205] -> w200
              tunnel: w197 -> [w203 w205]
              tunnel: w196 -> [w202 _]
              tunnel: w193 -> [w201 _]
              frame True {
                n66 = invoke class="VI" method="FP.Open"(reference=w202, error in=w203, "State"=w201) -> (error out=w204:errorcluster)  [unwired: 2 in, 4 out]
              }
              frame False {
              }
            }
          }
          frame "Minimize", "Minimized" {
            w206 = T1."Minimized" ("State")
            n67 = property class="VI"(reference=w212, error in=w211) -> (reference out=w209:refnum<vi>, error out=w210:errorcluster, "FP.State"=w208:T1)
            n68 = Not Equal?(x=w208, y=w206) -> (x != y?=w207:bool)
            n69 = case shown="True" w207 {
              tunnel: [w217 w218] -> w213
              tunnel: w210 -> [w216 w218]
              tunnel: w209 -> [w215 _]
              tunnel: w206 -> [w214 _]
              frame True {
                n70 = invoke class="VI" method="FP.Open"(reference=w215, error in=w216, "State"=w214) -> (error out=w217:errorcluster)  [unwired: 2 in, 4 out]
              }
              frame False {
              }
            }
          }
          frame "Maximize", "Maximized" {
            w219 = T1."Maximized" ("State")
            n71 = property class="VI"(reference=w225, error in=w224) -> (reference out=w222:refnum<vi>, error out=w223:errorcluster, "FP.State"=w221:T1)
            n72 = Not Equal?(x=w221, y=w219) -> (x != y?=w220:bool)
            n73 = case shown="True" w220 {
              tunnel: [w230 w231] -> w226
              tunnel: w223 -> [w229 w231]
              tunnel: w222 -> [w228 _]
              tunnel: w219 -> [w227 _]
              frame True {
                n74 = invoke class="VI" method="FP.Open"(reference=w228, error in=w229, "State"=w227) -> (error out=w230:errorcluster)  [unwired: 2 in, 4 out]
              }
              frame False {
              }
            }
          }
        }
        n75 = call <vilib>:"Add State(s) to Queue__JKI_lib_State_Machine.vi"("State(s) in (\"\")"=w166) -> ("States Out"=w165:string)  [unwired: 14 in]
      }
      frame "---------- Macro ----------" {
        # "Do not put any code in this frame.\n(It is a separator no-op. You can make a copy of this frame to create a new Macro frame)"
        n76 = call <vilib>:"Add State(s) to Queue__JKI_lib_State_Machine.vi"("State(s) in (\"\")"=w235) -> ("States Out"=w234:string)  [unwired: 14 in]
      }
      frame "Macro: Initialize" {
        # "Initialization Macro\n(This is called once, when the VI starts)"
        n77 = call <vilib>:"Add State(s) to Queue__JKI_lib_State_Machine.vi"("State(s) in Front (\"\")"="Data: Initialize\nInitialize Core Data\nUI: Initialize", "State(s) in (\"\")"=w240) -> ("States Out"=w239:string)  [unwired: 13 in]
      }
      frame "Macro: Exit" {
        # "Exit Macro\n(This is called once, when the VI exits)"
        n78 = Unbundle By Name(w247) -> ("Core.Close Panel on Exit?"=w246:bool)
        n79 = Select(t="UI: Front Panel State >> Close", s=w246, f="") -> (s? t:f=w243:string)
        n80 = call <vilib>:"Add State(s) to Queue__JKI_lib_State_Machine.vi"("State(s) in (\"\")"=w243, "State(s) at Back (\"\")"="Data: Cleanup\nExit") -> ("States Out"=w241:string)  [unwired: 13 in]
        n81 = call <vilib>:"Add State(s) to Queue__JKI_lib_State_Machine.vi"("State(s) in Front (\"\")"=w241, "State(s) in (\"\")"=w250) -> ("States Out"=w249:string)  [unwired: 13 in]
      }
      frame "---------- New Category ----------" {
        # "Template Separator\n(You can make a copy of, or modify, this frame)"
        n82 = call <vilib>:"Add State(s) to Queue__JKI_lib_State_Machine.vi"("State(s) in (\"\")"=w254) -> ("States Out"=w253:string)  [unwired: 14 in]
      }
      frame "New Category: 1" {
        # "Your code here.\n(You can make a copy of, or modify, this frame)"
        n83 = call <vilib>:"Add State(s) to Queue__JKI_lib_State_Machine.vi"("State(s) in (\"\")"=w258) -> ("States Out"=w257:string)  [unwired: 14 in]
      }
      frame "New Category: 2" {
        # "Your code here.\n(You can make a copy of, or modify, this frame)"
        n84 = call <vilib>:"Add State(s) to Queue__JKI_lib_State_Machine.vi"("State(s) in (\"\")"=w262) -> ("States Out"=w261:string)  [unwired: 14 in]
      }
      frame "---------- Test ----------" {
        # "Template Separator\n(You can make a copy of, or modify, this frame)"
        n85 = call <vilib>:"Add State(s) to Queue__JKI_lib_State_Machine.vi"("State(s) in (\"\")"=w266) -> ("States Out"=w265:string)  [unwired: 14 in]
      }
      frame "Test: Do Something" {
        n86 = call <vilib>:"Space Constant.vi"() -> ("String"=w273:string)
        n87 = Empty String/Path?(string/path=w268) -> (empty?=w272:bool)
        n88 = Concatenate Strings(w273, "from" ("string"), w273, w268) -> (w271:string)
        n89 = Select(t="", s=w272, f=w271) -> (s? t:f=w269:string)
        n90 = Concatenate Strings("\"Do Something\" excute" ("\"Do Something\" button pressed"), w269) -> (w267:string)
        "Status" <- w267
      }
      frame "Test: Do Something Else" {
        n91 = call <vilib>:"Space Constant.vi"() -> ("String"=w288:string)
        n92 = Empty String/Path?(string/path=w283) -> (empty?=w287:bool)
        n93 = Concatenate Strings(w288, "from" ("string"), w288, w283) -> (w286:string)
        n94 = Select(t="", s=w287, f=w286) -> (s? t:f=w284:string)
        n95 = Concatenate Strings("\"Do Something Else\" excute, para:" ("\"Do Something\" button pressed"), w281, w284) -> (w279:string)
        n96 = Fract/Exp String To Number(string=w281) -> (number=→"X":dbl)  [unwired: 3 in, 1 out]
        n97 = local write "Status"(w279) -> ()
      }
      frame "Test: Do Something Else and Wait for Reply" {
        n98 = call <vilib>:"Space Constant.vi"() -> ("String"=w304:string)
        n99 = Empty String/Path?(string/path=w299) -> (empty?=w303:bool)
        n100 = Concatenate Strings(w304, "from" ("string"), w304, w299) -> (w302:string)
        n101 = Select(t="", s=w303, f=w302) -> (s? t:f=w300:string)
        n102 = Concatenate Strings("\"Do Something Else and Wait for Reply\" excute, para:" ("\"Do Something\" button pressed"), w296, w300) -> (w298:string)
        n103 = Fract/Exp String To Number(string=w296) -> (number=w295:dbl)  [unwired: 3 in, 1 out]
        n104 = Random Number (0-1)() -> (number: 0 to 1=w294:dbl)
        n105 = local write "Status"(w298) -> ()
        n106 = local write "X"(w295) -> ()
        n107 = Number To Fractional String(number=w294) -> (F-format string=w293:string)  [unwired: 3 in]
      }
    }
  }
  "error out" <- w1
